vi "Hardware-DiffIOSetupCalPoints.vi"(11 "Diff I/O Setup":T1[](array[typedef])=[{"Mode"=enum."Pulse Width Modulation", "Capture Start [DBTDC]"=0.0, "Capture End [DBTDC]"=0.0, "Polarity"=FALSE, "Frequency [Hz]"=10.0, "Duty Cycle [%]"=1.0, "TDC Offset [CAD]"=0.0, "Window Start [DBTDC]"=0.0, "Window End [DBTDC]"=0.0, "Angles"=[{"Enable"=FALSE, "Location [DBTDC]"=0.0, "Duration [s]"=0.0}, {"Enable"=FALSE, "Location [DBTDC]"=0.0, "Duration [s]"=0.0}, {"Enable"=FALSE, "Location [DBTDC]"=0.0, "Duration [s]"=0.0}, {"Enable"=FALSE, "Location [DBTDC]"=0.0, "Duration [s]"=0.0}], "Skip Fire"=FALSE, "Skip Fire Index"=0}, {"Mode"=enum."Off", "Capture Start [DBTDC]"=0.0, "Capture End [DBTDC]"=0.0, "Polarity"=FALSE, "Frequency [Hz]"=0.0, "Duty Cycle [%]"=0.0, "TDC Offset [CAD]"=0.0, "Window Start [DBTDC]"=0.0, "Window End [DBTDC]"=0.0, "Angles"=[{"Enable"=FALSE, "Location [DBTDC]"=0.0, "Duration [s]"=0.0}, {"Enable"=FALSE, "Location [DBTDC]"=0.0, "Duration [s]"=0.0}, {"Enable"=FALSE, "Location [DBTDC]"=0.0, "Duration [s]"=0.0}, {"Enable"=FALSE, "Location [DBTDC]"=0.0, "Duration [s]"=0.0}], "Skip Fire"=FALSE, "Skip Fire Index"=0}, {"Mode"=enum."Off", "Capture Start [DBTDC]"=0.0, "Capture End [DBTDC]"=0.0, "Polarity"=FALSE, "Frequency [Hz]"=0.0, "Duty Cycle [%]"=0.0, "TDC Offset [CAD]"=0.0, "Window Start [DBTDC]"=0.0, "Window End [DBTDC]"=0.0, "Angles"=[{"Enable"=FALSE, "Location [DBTDC]"=0.0, "Duration [s]"=0.0}, {"Enable"=FALSE, "Location [DBTDC]"=0.0, "Duration [s]"=0.0}, {"Enable"=FALSE, "Location [DBTDC]"=0.0, "Duration [s]"=0.0}, {"Enable"=FALSE, "Location [DBTDC]"=0.0, "Duration [s]"=0.0}], "Skip Fire"=FALSE, "Skip Fire Index"=0}, {"Mode"=enum."Off", "Capture Start [DBTDC]"=0.0, "Capture End [DBTDC]"=0.0, "Polarity"=FALSE, "Frequency [Hz]"=0.0, "Duty Cycle [%]"=0.0, "TDC Offset [CAD]"=0.0, "Window Start [DBTDC]"=0.0, "Window End [DBTDC]"=0.0, "Angles"=[{"Enable"=FALSE, "Location [DBTDC]"=0.0, "Duration [s]"=0.0}, {"Enable"=FALSE, "Location [DBTDC]"=0.0, "Duration [s]"=0.0}, {"Enable"=FALSE, "Location [DBTDC]"=0.0, "Duration [s]"=0.0}, {"Enable"=FALSE, "Location [DBTDC]"=0.0, "Duration [s]"=0.0}], "Skip Fire"=FALSE, "Skip Fire Index"=0}, {"Mode"=enum."Off", "Capture Start [DBTDC]"=0.0, "Capture End [DBTDC]"=0.0, "Polarity"=FALSE, "Frequency [Hz]"=0.0, "Duty Cycle [%]"=0.0, "TDC Offset [CAD]"=0.0, "Window Start [DBTDC]"=0.0, "Window End [DBTDC]"=0.0, "Angles"=[{"Enable"=FALSE, "Location [DBTDC]"=0.0, "Duration [s]"=0.0}, {"Enable"=FALSE, "Location [DBTDC]"=0.0, "Duration [s]"=0.0}, {"Enable"=FALSE, "Location [DBTDC]"=0.0, "Duration [s]"=0.0}, {"Enable"=FALSE, "Location [DBTDC]"=0.0, "Duration [s]"=0.0}], "Skip Fire"=FALSE, "Skip Fire Index"=0}, {"Mode"=enum."Off", "Capture Start [DBTDC]"=0.0, "Capture End [DBTDC]"=0.0, "Polarity"=FALSE, "Frequency [Hz]"=0.0, "Duty Cycle [%]"=0.0, "TDC Offset [CAD]"=0.0, "Window Start [DBTDC]"=0.0, "Window End [DBTDC]"=0.0, "Angles"=[{"Enable"=FALSE, "Location [DBTDC]"=0.0, "Duration [s]"=0.0}, {"Enable"=FALSE, "Location [DBTDC]"=0.0, "Duration [s]"=0.0}, {"Enable"=FALSE, "Location [DBTDC]"=0.0, "Duration [s]"=0.0}, {"Enable"=FALSE, "Location [DBTDC]"=0.0, "Duration [s]"=0.0}], "Skip Fire"=FALSE, "Skip Fire Index"=0}, {"Mode"=enum."Off", "Capture Start [DBTDC]"=0.0, "Capture End [DBTDC]"=0.0, "Polarity"=FALSE, "Frequency [Hz]"=0.0, "Duty Cycle [%]"=0.0, "TDC Offset [CAD]"=0.0, "Window Start [DBTDC]"=0.0, "Window End [DBTDC]"=0.0, "Angles"=[{"Enable"=FALSE, "Location [DBTDC]"=0.0, "Duration [s]"=0.0}, {"Enable"=FALSE, "Location [DBTDC]"=0.0, "Duration [s]"=0.0}, {"Enable"=FALSE, "Location [DBTDC]"=0.0, "Duration [s]"=0.0}, {"Enable"=FALSE, "Location [DBTDC]"=0.0, "Duration [s]"=0.0}], "Skip Fire"=FALSE, "Skip Fire Index"=0}, {"Mode"=enum."Off", "Capture Start [DBTDC]"=0.0, "Capture End [DBTDC]"=0.0, "Polarity"=FALSE, "Frequency [Hz]"=0.0, "Duty Cycle [%]"=0.0, "TDC Offset [CAD]"=0.0, "Window Start [DBTDC]"=0.0, "Window End [DBTDC]"=0.0, "Angles"=[{"Enable"=FALSE, "Location [DBTDC]"=0.0, "Duration [s]"=0.0}, {"Enable"=FALSE, "Location [DBTDC]"=0.0, "Duration [s]"=0.0}, {"Enable"=FALSE, "Location [DBTDC]"=0.0, "Duration [s]"=0.0}, {"Enable"=FALSE, "Location [DBTDC]"=0.0, "Duration [s]"=0.0}], "Skip Fire"=FALSE, "Skip Fire Index"=0}] {"Skip Fire Index" max=7; "Angles"."Duration [s]" format="%#_3p"; "Frequency [Hz]" format="%#_3p"}) -> (3 "Diff I/O Setup":T1[](array[typedef])=[{"Mode"=enum."Pulse Width Modulation", "Capture Start [DBTDC]"=0.0, "Capture End [DBTDC]"=0.0, "Polarity"=FALSE, "Frequency [Hz]"=10.0, "Duty Cycle [%]"=1.0, "TDC Offset [CAD]"=0.0, "Window Start [DBTDC]"=0.0, "Window End [DBTDC]"=0.0, "Angles"=[{"Enable"=FALSE, "Location [DBTDC]"=0.0, "Duration [s]"=0.0}, {"Enable"=FALSE, "Location [DBTDC]"=0.0, "Duration [s]"=0.0}, {"Enable"=FALSE, "Location [DBTDC]"=0.0, "Duration [s]"=0.0}, {"Enable"=FALSE, "Location [DBTDC]"=0.0, "Duration [s]"=0.0}], "Skip Fire"=FALSE, "Skip Fire Index"=0}, {"Mode"=enum."Off", "Capture Start [DBTDC]"=0.0, "Capture End [DBTDC]"=0.0, "Polarity"=FALSE, "Frequency [Hz]"=0.0, "Duty Cycle [%]"=0.0, "TDC Offset [CAD]"=0.0, "Window Start [DBTDC]"=0.0, "Window End [DBTDC]"=0.0, "Angles"=[{"Enable"=FALSE, "Location [DBTDC]"=0.0, "Duration [s]"=0.0}, {"Enable"=FALSE, "Location [DBTDC]"=0.0, "Duration [s]"=0.0}, {"Enable"=FALSE, "Location [DBTDC]"=0.0, "Duration [s]"=0.0}, {"Enable"=FALSE, "Location [DBTDC]"=0.0, "Duration [s]"=0.0}], "Skip Fire"=FALSE, "Skip Fire Index"=0}, {"Mode"=enum."Off", "Capture Start [DBTDC]"=0.0, "Capture End [DBTDC]"=0.0, "Polarity"=FALSE, "Frequency [Hz]"=0.0, "Duty Cycle [%]"=0.0, "TDC Offset [CAD]"=0.0, "Window Start [DBTDC]"=0.0, "Window End [DBTDC]"=0.0, "Angles"=[{"Enable"=FALSE, "Location [DBTDC]"=0.0, "Duration [s]"=0.0}, {"Enable"=FALSE, "Location [DBTDC]"=0.0, "Duration [s]"=0.0}, {"Enable"=FALSE, "Location [DBTDC]"=0.0, "Duration [s]"=0.0}, {"Enable"=FALSE, "Location [DBTDC]"=0.0, "Duration [s]"=0.0}], "Skip Fire"=FALSE, "Skip Fire Index"=0}, {"Mode"=enum."Off", "Capture Start [DBTDC]"=0.0, "Capture End [DBTDC]"=0.0, "Polarity"=FALSE, "Frequency [Hz]"=0.0, "Duty Cycle [%]"=0.0, "TDC Offset [CAD]"=0.0, "Window Start [DBTDC]"=0.0, "Window End [DBTDC]"=0.0, "Angles"=[{"Enable"=FALSE, "Location [DBTDC]"=0.0, "Duration [s]"=0.0}, {"Enable"=FALSE, "Location [DBTDC]"=0.0, "Duration [s]"=0.0}, {"Enable"=FALSE, "Location [DBTDC]"=0.0, "Duration [s]"=0.0}, {"Enable"=FALSE, "Location [DBTDC]"=0.0, "Duration [s]"=0.0}], "Skip Fire"=FALSE, "Skip Fire Index"=0}, {"Mode"=enum."Off", "Capture Start [DBTDC]"=0.0, "Capture End [DBTDC]"=0.0, "Polarity"=FALSE, "Frequency [Hz]"=0.0, "Duty Cycle [%]"=0.0, "TDC Offset [CAD]"=0.0, "Window Start [DBTDC]"=0.0, "Window End [DBTDC]"=0.0, "Angles"=[{"Enable"=FALSE, "Location [DBTDC]"=0.0, "Duration [s]"=0.0}, {"Enable"=FALSE, "Location [DBTDC]"=0.0, "Duration [s]"=0.0}, {"Enable"=FALSE, "Location [DBTDC]"=0.0, "Duration [s]"=0.0}, {"Enable"=FALSE, "Location [DBTDC]"=0.0, "Duration [s]"=0.0}], "Skip Fire"=FALSE, "Skip Fire Index"=0}, {"Mode"=enum."Off", "Capture Start [DBTDC]"=0.0, "Capture End [DBTDC]"=0.0, "Polarity"=FALSE, "Frequency [Hz]"=0.0, "Duty Cycle [%]"=0.0, "TDC Offset [CAD]"=0.0, "Window Start [DBTDC]"=0.0, "Window End [DBTDC]"=0.0, "Angles"=[{"Enable"=FALSE, "Location [DBTDC]"=0.0, "Duration [s]"=0.0}, {"Enable"=FALSE, "Location [DBTDC]"=0.0, "Duration [s]"=0.0}, {"Enable"=FALSE, "Location [DBTDC]"=0.0, "Duration [s]"=0.0}, {"Enable"=FALSE, "Location [DBTDC]"=0.0, "Duration [s]"=0.0}], "Skip Fire"=FALSE, "Skip Fire Index"=0}, {"Mode"=enum."Off", "Capture Start [DBTDC]"=0.0, "Capture End [DBTDC]"=0.0, "Polarity"=FALSE, "Frequency [Hz]"=0.0, "Duty Cycle [%]"=0.0, "TDC Offset [CAD]"=0.0, "Window Start [DBTDC]"=0.0, "Window End [DBTDC]"=0.0, "Angles"=[{"Enable"=FALSE, "Location [DBTDC]"=0.0, "Duration [s]"=0.0}, {"Enable"=FALSE, "Location [DBTDC]"=0.0, "Duration [s]"=0.0}, {"Enable"=FALSE, "Location [DBTDC]"=0.0, "Duration [s]"=0.0}, {"Enable"=FALSE, "Location [DBTDC]"=0.0, "Duration [s]"=0.0}], "Skip Fire"=FALSE, "Skip Fire Index"=0}, {"Mode"=enum."Off", "Capture Start [DBTDC]"=0.0, "Capture End [DBTDC]"=0.0, "Polarity"=FALSE, "Frequency [Hz]"=0.0, "Duty Cycle [%]"=0.0, "TDC Offset [CAD]"=0.0, "Window Start [DBTDC]"=0.0, "Window End [DBTDC]"=0.0, "Angles"=[{"Enable"=FALSE, "Location [DBTDC]"=0.0, "Duration [s]"=0.0}, {"Enable"=FALSE, "Location [DBTDC]"=0.0, "Duration [s]"=0.0}, {"Enable"=FALSE, "Location [DBTDC]"=0.0, "Duration [s]"=0.0}, {"Enable"=FALSE, "Location [DBTDC]"=0.0, "Duration [s]"=0.0}], "Skip Fire"=FALSE, "Skip Fire Index"=0}] {"Skip Fire Index" max=7; "Angles"."Duration [s]" format="%#_3p"; "Frequency [Hz]" format="%#_3p"})   [LabVIEW 2016, in "DSI-RT.lvlib"]
uses:
  DSI-RT.lvlib
  <vilib>/Powertrain Controls/Device Drivers/DCM/Diff IO/RT/Setup.ctl
  <vilib>/Powertrain Controls/Device Drivers/DCM/Diff IO/FPGA/Mode.ctl
  <vilib>/Powertrain Controls/Device Drivers/DCM/Diff IO/RT/Angle Control.ctl
  <vilib>/addons/Software Calibration Management/xSCM/CalPoint.xnode
  <vilib>/addons/Software Calibration Management/xSCM/ni_scm.dll
  <vilib>/Powertrain Controls/Device Drivers/DCM/Diff IO/RT/DCM - RT - Diff IO.lvlib
  <vilib>/Powertrain Controls/Device Drivers/DCM/Diff IO/FPGA/DCM - FPGA - Diff IO.lvlib
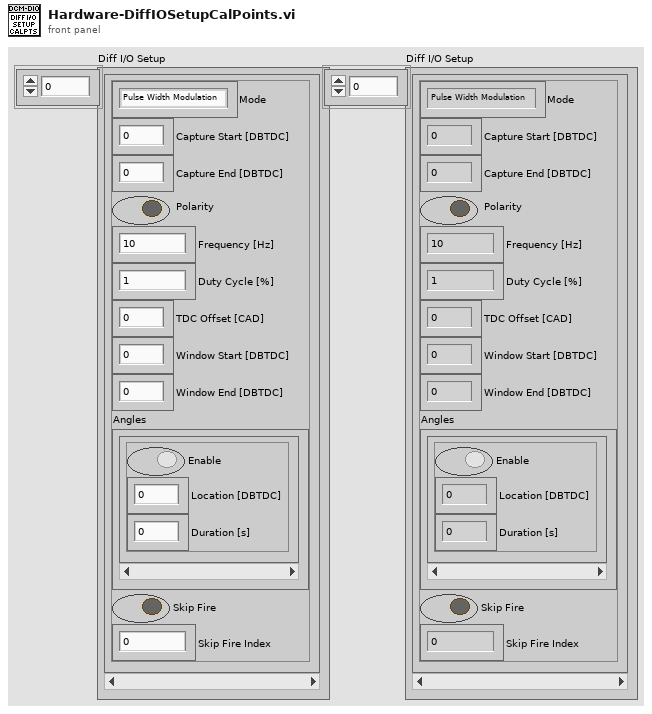
[diagram p1: front panel]
types:
  T1 = typedef "DCM - RT - Diff IO.lvlib/Setup.ctl" = cluster{"Mode":T2, "Capture Start [DBTDC]":sgl, "Capture End [DBTDC]":sgl, "Polarity":bool, "Frequency [Hz]":sgl, "Duty Cycle [%]":sgl, "TDC Offset [CAD]":sgl, "Window Start [DBTDC]":sgl, "Window End [DBTDC]":sgl, "Angles":T3[], "Skip Fire":bool, "Skip Fire Index":u8}
  T2 = typedef "DCM - FPGA - Diff IO.lvlib/Mode.ctl" = enum8{"Off", "Input", "Pulse Width Modulation", "Engine Position Tracking", "Serial Out 1", "Serial Out 2"}
  T3 = typedef "DCM - RT - Diff IO.lvlib/Angle Control.ctl" = cluster{"Enable":bool, "Location [DBTDC]":sgl, "Duration [s]":sgl}
  T4 = cluster{"Mode":enum8{"Off", "Input", "Pulse Width Modulation", "Engine Position Tracking"}, "Capture Start [DBTDC]":sgl, "Capture End [DBTDC]":sgl, "Polarity":bool, "Frequency [Hz]":sgl, "Duty Cycle [%]":sgl, "TDC Offset [CAD]":sgl, "Window Start [DBTDC]":sgl, "Window End [DBTDC]":sgl, "Angles":cluster{"Enable":bool, "Location [DBTDC]":sgl, "Duration [s]":sgl}[], "Skip Fire":bool, "Skip Fire Index":u8}[]
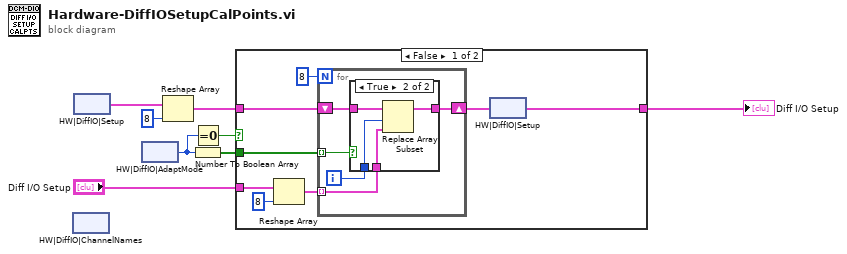
[diagram p0: block diagram]
diagram:
  n1 = xnode "HW|DiffIO|ChannelNames"() -> ()  [unwired: 1 out]
  n2 = xnode "HW|DiffIO|Setup"() -> ("Value"=w1:T4)
  n3 = xnode "HW|DiffIO|AdaptMode"() -> ("Value"=w5:u32)
  n4 = Reshape Array(w1, 8 ("dimension size")) -> (w8:T4)
  n5 = Equal To 0?(x=w5) -> (x = 0?=w4:bool)
  n6 = Number To Boolean Array(number=w5) -> (Boolean array=w6:bool[])
  n7 = case shown="False" w4 {
    tunnel: w8 -> [w15 w31]
    tunnel: [w9 w31] -> w2
    tunnel: w6 -> [w13 _]
    tunnel: "Diff I/O Setup" -> [w10 _]
    frame False {
      n8 = Reshape Array(w10, 8 ("dimension size")) -> (w11:T1[])
      n9 = for {
        N: 8 -> [_]
        tunnel: w13 -> [w21] mode=indexing
        shift-right: [w24] -> w9
        shift-left: w15 -> [w25]
        tunnel: w11 -> [w22] mode=indexing
        i -> [w23]
        n10 = case shown="True" w21 {
          tunnel: w25 -> [w26 w30]
          tunnel: [w26 w29] -> w24
          tunnel: w23 -> [_ w28]
          tunnel: w22 -> [_ w27]
          frame False {
          }
          frame True {
            n11 = Replace Array Subset(array=w30, new element=w27, index=w28) -> (w29:T4)
          }
        }
      }
      n12 = xnode "HW|DiffIO|Setup"("Value"=w9) -> ()
    }
    frame True {
    }
  }
  "Diff I/O Setup" <- w2
